vi "Online Pitch Shifting.vi"() -> ()   [LabVIEW 2023]
doc: "This example shows how to configure a sound card device, continuously acquire and play sound data, and shift the pitch of a normal speech with the TFA Online Gabor Transform VI and Online Gabor Expansion VI.\n\n<b>Instructions:</b>\n1) Run this VI.\n2) Adjust the <b>Pitch multiplier</b>.\n3) Speak into the microphone.\n4) Listen to the output pitch shifted speech.\n5) Browse the Block Diagram of this example to learn how to use the TFA Online Gabor Transform VI and TFA Online Gabor Expansion VI."
uses:
  <vilib>/sound2/lvsound2.llb/Sound Data Format.ctl
  <vilib>/sound2/lvsound2.llb/Sound Input Read (DBL).vi
  <vilib>/addons/Time Frequency Analysis/Transform.llb/TFA Online Gabor Transform (Real).vi
  <vilib>/addons/Time Frequency Analysis/Transform.llb/TFA Online Gabor Expansion (Real).vi
  <vilib>/Analysis/2dsp.llb/Resample (constant to constant,single -channel).vi
  <vilib>/sound2/lvsound2.llb/Sound Output Write (DBL Single).vi
  <vilib>/addons/_Advanced Signal Processing/NI_AdvSigProcTFA.lvlib
  <vilib>/Analysis/NI_AALPro.lvlib
panel:
  in  "Pitch multiplier":dbl(slide)=1.0 scale=0.5..2.0
  out "Pitch Shifted Speech":dbl[](graph)
  out "aspt-left-top":bool
  in  "Stop":bool
  out "Original Speech":dbl[](graph)
  # "Overview: Shows how to configure a sound card device, continuously acquire and play sound data, and shift the pitch of a normal speech with the TFA Online Gabor Transform VI and Online Gabor Expansion VI.\nRequirements: LabVIEW Full Development System, Advanced Signal Processing Toolkit, Microphone\nInstructions: \n1. Run this VI.\n2. Adjust the Pitch multiplier.\n3. Speak into the microphone.\n4. Listen to the output pitch shifted speech.\n5. Browse the block diagram of this example to learn how to use the TFA Online Gabor Transform VI and TFA Online Gabor Expansion VI.\n6. Click Stop to stop the VI."
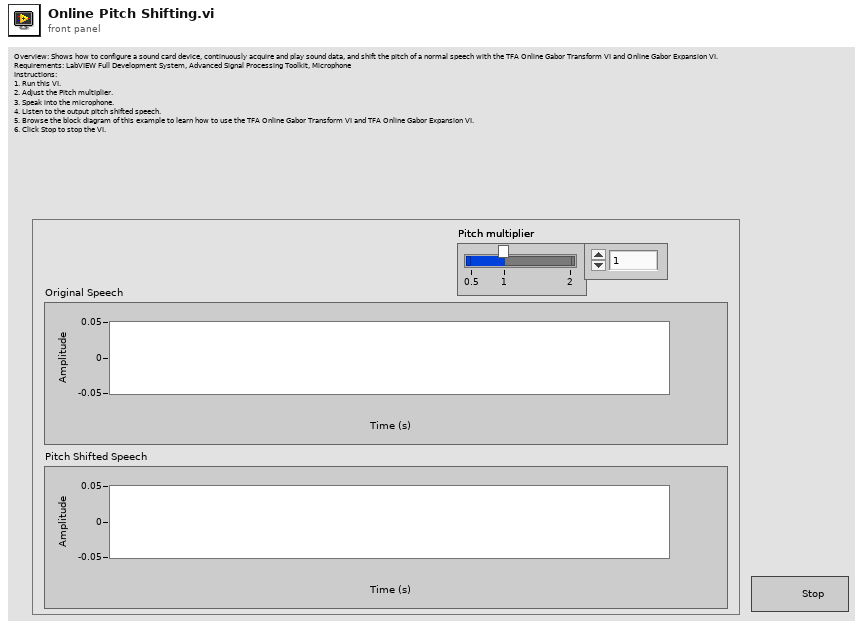
[diagram p1: front panel]
types:
  T1 = typedef "Sound Data Format.ctl" = cluster{"sample rate (S/s)":dbl, "number of channels":i32, "bits per sample":i32}
  T2 = typedef "Sound Input Task ID.ctl" = u32
  T3 = typedef "Sound Output Task ID.ctl" = u32
  T4 = cluster{"synthesis window":dbl[], "dM (time steps)":i32, "N (frequency bins)":i32}
  T5 = cluster{"analysis window":dbl[], "dM (time steps)":i32, "N (frequency bins)":i32}
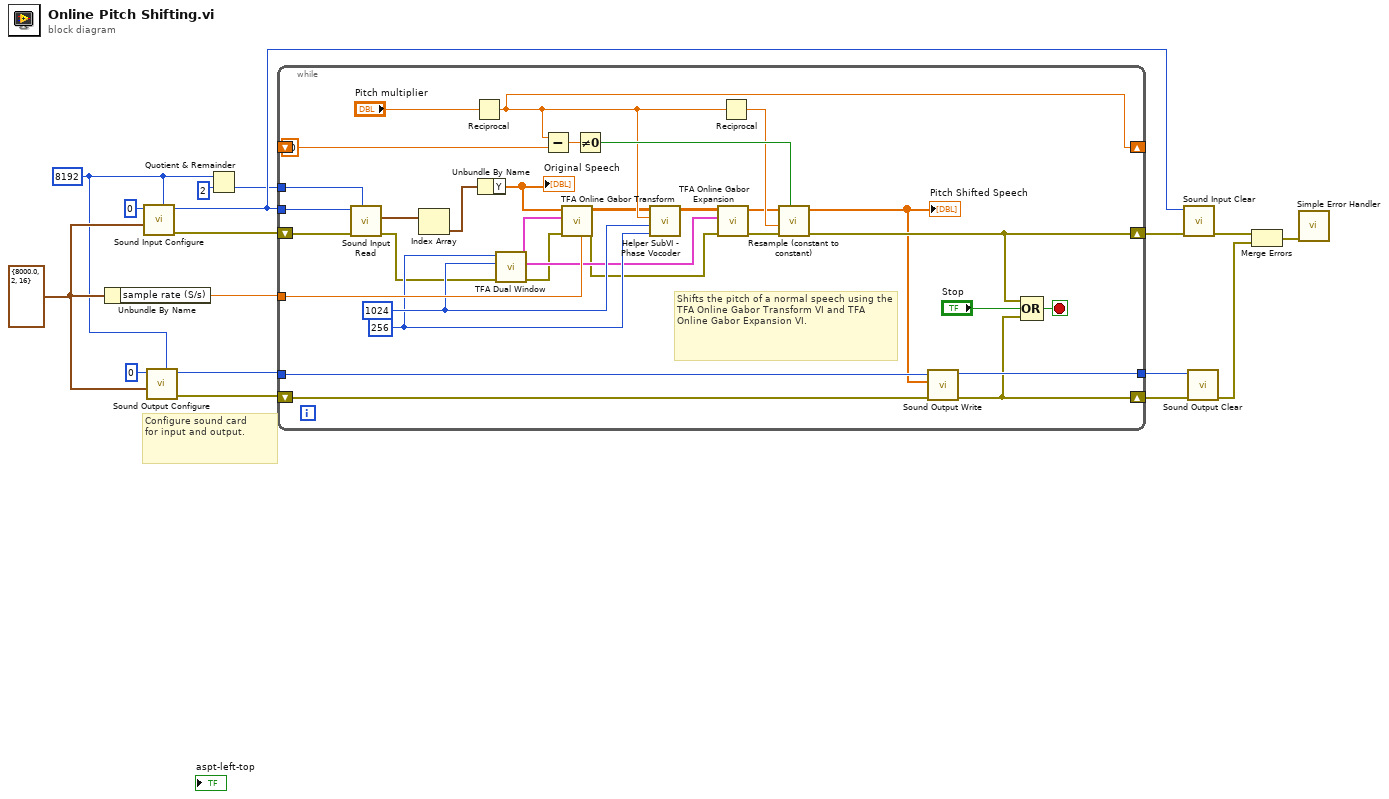
[diagram p0: block diagram]
diagram:
  w3 = 8192 ("number of samples/ch")
  w13 = T1 {"sample rate (S/s)"=8000.0, "number of channels"=2, "bits per sample"=16} ("sound format")
  # "Configure sound card\nfor input and output."
  n1 = Unbundle By Name(w13) -> ("sample rate (S/s)"=w12:dbl)
  n2 = call <vilib>:"Sound Input Configure.vi"("number of samples/ch"=w3, "sound format"=w13, "device ID"=u32 0 ("device (0)")) -> ("error out"=w6:errorcluster, "task ID"=w7:T2)  [unwired: 7 in]
  n3 = call <vilib>:"Sound Output Configure.vi"("number of samples/ch"=w3, "sound format"=w13, "device ID"=u32 0 ("device (0)")) -> ("error out"=w4:errorcluster, "task ID"=w5:T3)  [unwired: 7 in]
  n4 = Quotient & Remainder(x=w3, y=2) -> (floor(x/y)=w1:i32)  [unwired: 1 out]
  n5 = while {
    tunnel: w7 -> [w50]
    tunnel: w5 -> [w32]
    tunnel: [w48] -> w9
    shift-right: [w37] -> w8
    shift-left: w4 -> [w31]
    tunnel: w12 -> [w41]
    shift-right: [w40] -> _
    shift-left: 0.0 -> [w46]
    shift-right: [w36] -> w10
    shift-left: w6 -> [w49]
    tunnel: w1 -> [w20]
    stop <- w47 stop-if-true
    w38 = 256 ("hop")
    w39 = 1024 ("N")
    # "Shifts the pitch of a normal speech using the TFA Online Gabor Transform VI and TFA Online Gabor Expansion VI."
    n6 = call-poly <vilib>:"Sound Input Read.vi"("number of samples/ch"=w20, "error in (no error)"=w49, "task ID"=w50) -> ("error out"=w35:errorcluster, "data"=w30:waveform(dbl)[])  [unwired: 6 in, 1 out]
    n7 = Index Array(array=w30) -> (element=w33:waveform(dbl))  [unwired: 1 in]
    n8 = Reciprocal(x="Pitch multiplier") -> (1/x=w40:dbl)
    n9 = Unbundle By Name(w33) -> ("Y"=w21:dbl[])
    "Original Speech" <- w21
    n10 = call <vilib>:"TFA Dual Window.vi"("error in (no error)"=w35, "N (frequency bins)"=w39, "dM (time steps)"=w38) -> ("error out"=w22:errorcluster, "synthesis info"=w28:T4, "analysis info"=w29:T5)  [unwired: 1 in, 5 out]
    n11 = Subtract(x=w40, y=w46) -> (x-y=w45:dbl)
    n12 = call-poly <vilib>:"TFA Online Gabor Transform.vi"("sampling rate"=w41, "error in (no error)"=w22, "transform info"=w29, "signal"=w21) -> ("error out"=w24:errorcluster, "Gabor coef"=w27:cdb[][])  [unwired: 6 out]
    n13 = Not Equal To 0?(x=w45) -> (x != 0?=w42:bool)
    n14 = call "Helper SubVI - Phase Vocoder.vi"("hop"=w38, "N"=w39, "squeeze"=w40, "STFT coefficients in"=w27) -> ("STFT coefficients out"=w26:cdb[][])  [unwired: 7 out]
    n15 = call-poly <vilib>:"TFA Online Gabor Expansion.vi"("error in (no error)"=w24, "expansion info"=w28, "Gabor coef"=w26) -> ("error out"=w23:errorcluster, "signal"=w25:dbl[])  [unwired: 7 out]
    n16 = Reciprocal(x=w40) -> (1/x=w34:dbl)
    n17 = call-poly <vilib>:"Resample (constant to constant).vi"("reset?"=w42, "error in (no error)"=w23, "dt"=w34, "X"=w25) -> ("error out"=w36:errorcluster, "Y"=w19:dbl[])  [unwired: 3 in, 3 out]
    "Pitch Shifted Speech" <- w19
    n18 = call-poly <vilib>:"Sound Output Write.vi"("error in (no error)"=w31, "data"=w19, "task ID"=w32) -> ("error out"=w37:errorcluster, "task ID out"=w48:T3)  [unwired: 7 in]
    n19 = Compound Arithmetic op=OR(w36, "Stop", w37) -> (w47:bool)
  }
  n20 = call <vilib>:"Sound Input Clear.vi"("error in (no error)"=w10, "task ID"=w7) -> ("error out"=w16:errorcluster)  [unwired: 9 in]
  n21 = call <vilib>:"Sound Output Clear.vi"("error in (no error)"=w8, "task ID"=w9) -> ("error out"=w15:errorcluster)  [unwired: 9 in]
  n22 = Merge Errors(w16, w15) -> (w14:errorcluster)
  n23 = call <vilib>:"Simple Error Handler.vi"("error in (no error)"=w14) -> ()  [unwired: 4 in, 5 out]
